vi "ExampleVI.vi"() -> ()   [LabVIEW 2024]
uses:
  DeconEngineClass/LaguerreDeconEngineClass.lvclass
  DeconEngineClass/LaguerreDeconEngineClass.lvclass/LaguerreDeconEngineClass.ctl
  <vilib>/Analysis/baseanly.llb/Mean (DBL).vi
  <vilib>/Utility/file.llb/Read Delimited Spreadsheet (DBL).vi
  <vilib>/Analysis/NI_AALBase.lvlib
panel:
  out "Histogram Graph":T1(graph)
  out "Lifetime Graph":dbl[](graph)
  out "iRF shift":dbl
  out "RMSE":dbl[](array[numeric])
  out "R square":dbl[](array[numeric])
  out "SSE":dbl[](array[numeric])
  in  "dataLength":i32=680
  out "iRF size(s)":i32
  out "data Matrix Szie":T2
  in  "plot index (row)":i32=45
  out "Decay Graph":dbl[][](graph)
  out "Computer time Graph":dbl[](graph)
  out "data Length":i32
  out "Waveform Graph":dbl[][](graph)
  out "alpha value":dbl
  in  "LaguerreDeconLib.lvlib:LaguerreDeconClass.lvclass":refnum<class "LaguerreDeconEngineClass.lvclass">
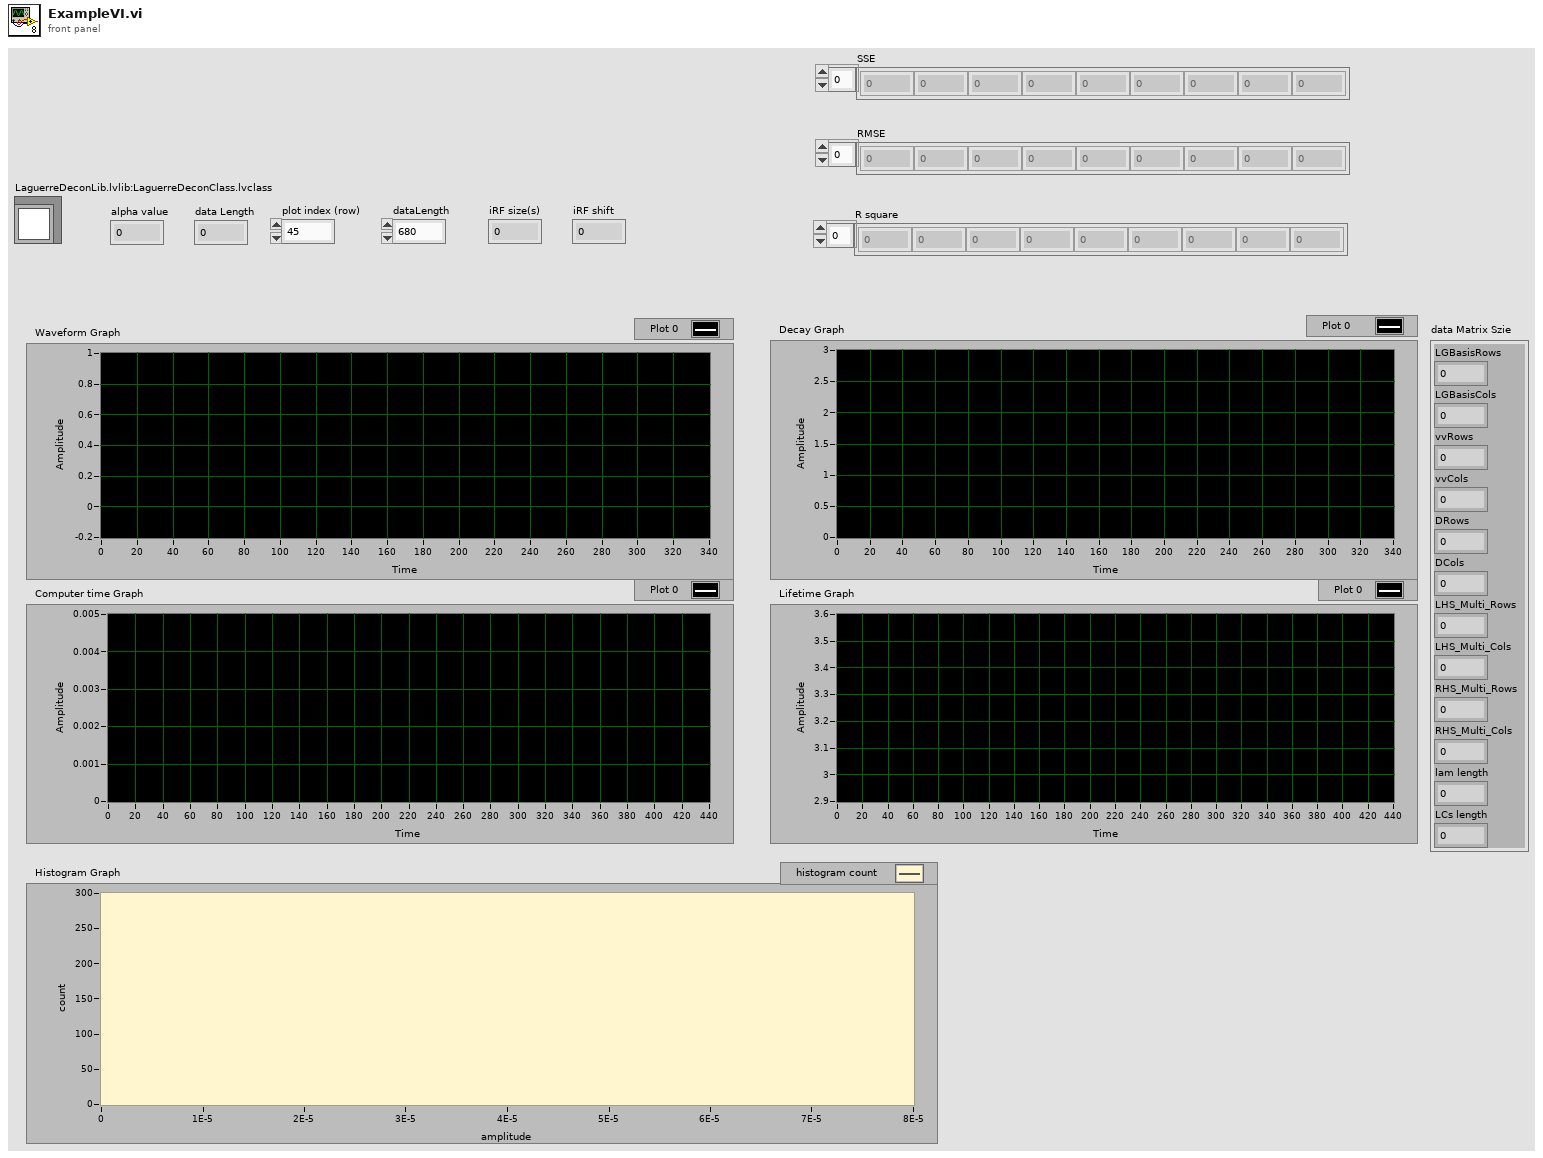
[diagram p1: front panel]
types:
  T1 = cluster{"X Values":dbl[], "Histogram: h(x)":i32[]}
  T2 = cluster{"LGBasisRows":u32, "LGBasisCols":u32, "vvRows":u32, "vvCols":u32, "DRows":u32, "DCols":u32, "LHS_Multi_Rows":u32, "LHS_Multi_Cols":u32, "RHS_Multi_Rows":u32, "RHS_Multi_Cols":u32, "lam length":u32, "LCs length":u32}
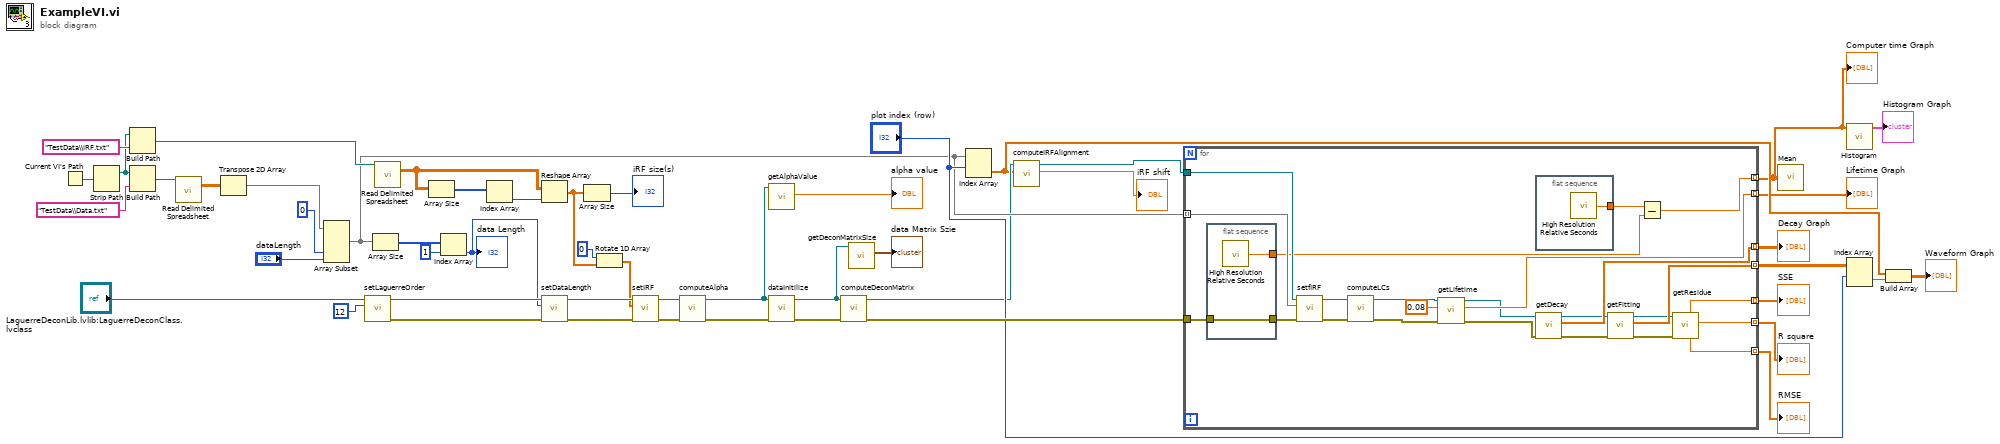
[diagram p0: block diagram]
diagram:
  n1 = Current VI's Path() -> (path=w22:path)
  n2 = Strip Path(path=w22) -> (stripped path=w18:path)  [unwired: 1 out]
  n3 = Build Path(base path=w18, name or relative path="TestData\\iRF.txt") -> (appended path=w17:path)
  n4 = Build Path(base path=w18, name or relative path="TestData\\Data.txt") -> (appended path=w20:path)
  n5 = call-poly <vilib>:"Read Delimited Spreadsheet.vi"("file path (dialog if empty)"=w20) -> ("all rows"=w35:dbl[][])  [unwired: 9 in, 5 out]
  n6 = Transpose 2D Array(2D array=w35) -> (transposed array=w33:dbl[][])
  n7 = Array Subset(array=w33, index (col)=0 ("index"), length (col)="dataLength") -> (w11:dbl[][])  [unwired: 2 in]
  n8 = call "setLaguerreOrder.vi"("LaguerreOrder"=u64 12, "LaguerreDeconClass in"="LaguerreDeconLib.lvlib:LaguerreDeconClass.lvclass") -> ("error out"=w46:errorcluster, "LaguerreDeconClass out"=w47:refnum<class "LaguerreDeconEngineClass.lvclass">)  [unwired: 8 in]
  n9 = Array Size(array=w11) -> (size(s)=w37:i32[])
  n10 = call-poly <vilib>:"Read Delimited Spreadsheet.vi"("file path (dialog if empty)"=w17) -> ("all rows"=w50:dbl[][])  [unwired: 9 in, 5 out]
  n11 = Array Size(array=w50) -> (size(s)=w51:i32[])
  n12 = Index Array(array=w37, index=1) -> (element=w36:i32)
  "data Length" <- w36
  n13 = Index Array(array=w51) -> (element=w40:i32)  [unwired: 1 in]
  n14 = Reshape Array(w50, w40) -> (w9:dbl[])
  n15 = call "setDataLength.vi"("error in (no error)"=w46, "dataLength"=w36, "LaguerreDeconClass in"=w47) -> ("error out"=w44:errorcluster, "LaguerreDeconClass out"=w45:refnum<class "LaguerreDeconEngineClass.lvclass">)  [unwired: 7 in]
  n16 = Array Size(array=w9) -> (size(s)=→"iRF size(s)":i32)
  n17 = Rotate 1D Array(1:w9, 2:0 ("n")) -> (0:w8:dbl[])
  n18 = call "setIRF.vi"("error in (no error)"=w44, "iRF"=w8, "LaguerreDeconClass in"=w45) -> ("error out"=w42:errorcluster, "LaguerreDeconClass out"=w43:refnum<class "LaguerreDeconEngineClass.lvclass">)  [unwired: 7 in]
  n19 = call "computeAlpha.vi"("error in (no error)"=w42, "LaguerreDeconClass in"=w43) -> ("error out"=w41:errorcluster, "LaguerreDeconClass out"=w30:refnum<class "LaguerreDeconEngineClass.lvclass">)  [unwired: 8 in]
  n20 = call "getAlphaValue.vi"("LaguerreDeconClass in"=w30) -> ("alpha value"=→"alpha value":dbl)  [unwired: 8 in, 2 out]
  n21 = call "dataInitilize.vi"("error in (no error)"=w41, "LaguerreDeconClass in"=w30) -> ("error out"=w39:errorcluster, "LaguerreDeconClass out"=w25:refnum<class "LaguerreDeconEngineClass.lvclass">)  [unwired: 8 in]
  n22 = call "computeDeconMatrix.vi"("error in (no error)"=w39, "LaguerreDeconClass in"=w25) -> ("error out"=w38:errorcluster, "LaguerreDeconClass out"=w10:refnum<class "LaguerreDeconEngineClass.lvclass">)  [unwired: 8 in]
  n23 = call "getDeconMatrixSize.vi"("LaguerreDeconClass in"=w25) -> ("data Matrix Szie"=→"data Matrix Szie":T2)  [unwired: 8 in, 2 out]
  n24 = Index Array(array=w11, index (row)="plot index (row)") -> (element=w5:dbl[])  [unwired: 1 in]
  n25 = call "computeIRFAlignment.vi"("fIRF temp"=w5, "LaguerreDeconEngineClass in"=w10) -> ("iRF shift"=→"iRF shift":dbl, "LaguerreDeconEngineClass out"=w4:refnum<class "LaguerreDeconEngineClass.lvclass">)  [unwired: 7 in, 1 out]
  n26 = for {
    tunnel: w4 -> [w70]
    tunnel: w38 -> [w58]
    tunnel: w11 -> [w68] mode=indexing
    tunnel: [w74] -> w2 mode=indexing
    tunnel: [w73] -> w31 mode=indexing
    tunnel: [w71] -> w28 mode=indexing
    tunnel: [w65] -> w14 mode=indexing
    tunnel: [w64] -> w13 mode=indexing
    tunnel: [w63] -> w12 mode=indexing
    tunnel: [w62] -> w3 mode=indexing
    n27 = flat-sequence {
      tunnel: [w77] -> w60
      tunnel: w58 -> [w76]
      tunnel: [w76] -> w57
      frame #0 {
        n28 = call <vilib>:"High Resolution Relative Seconds.vi"() -> ("relative seconds"=w77:dbl)
      }
    }
    n29 = call "setfIRF.vi"("error in (no error)"=w57, "fIRF"=w68, "LaguerreDeconEngineClass in"=w70) -> ("error out"=w59:errorcluster, "LaguerreDeconEngineClass out"=w69:refnum<class "LaguerreDeconEngineClass.lvclass">)  [unwired: 7 in]
    n30 = call "computeLCs.vi"("error in (no error)"=w59, "LaguerreDeconClass in"=w69) -> ("error out"=w55:errorcluster, "LaguerreDeconClass out"=w54:refnum<class "LaguerreDeconEngineClass.lvclass">)  [unwired: 8 in]
    n31 = call "getLifetime.vi"("error in (no error)"=w55, "dt (ns)"=0.08, "LaguerreDeconEngineClass in"=w54) -> ("error out"=w52:errorcluster, "lifetime (ns)"=w62:dbl, "LaguerreDeconEngineClass out"=w53:refnum<class "LaguerreDeconEngineClass.lvclass">)  [unwired: 6 in]
    n32 = flat-sequence {
      tunnel: [w78] -> w75
      frame #0 {
        n33 = call <vilib>:"High Resolution Relative Seconds.vi"() -> ("relative seconds"=w78:dbl)
      }
    }
    n34 = call "getDecay.vi"("error in (no error)"=w52, "LaguerreDeconClass in"=w53) -> ("error out"=w56:errorcluster, "Decay"=w73:dbl[], "LaguerreDeconClass out"=w72:refnum<class "LaguerreDeconEngineClass.lvclass">)  [unwired: 7 in]
    n35 = call "getFitting.vi"("error in (no error)"=w56, "LaguerreDeconEngineClass in"=w72) -> ("error out"=w66:errorcluster, "Fitting"=w71:dbl[], "LaguerreDeconEngineClass out"=w67:refnum<class "LaguerreDeconEngineClass.lvclass">)  [unwired: 7 in]
    n36 = Subtract(x=w75, y=w60) -> (x-y=w74:dbl)
    n37 = call "getResidue.vi"("error in (no error)"=w66, "LaguerreDeconEngineClass in"=w67) -> ("R-square"=w64:dbl, "RMSE"=w63:dbl, "SSE"=w65:dbl)  [unwired: 5 in, 2 out]
  }
  "Computer time Graph" <- w2
  "Decay Graph" <- w31
  "SSE" <- w14
  "R square" <- w13
  "RMSE" <- w12
  "Lifetime Graph" <- w3
  n38 = call-poly <vilib>:"Mean.vi"("X"=w2) -> ()  [unwired: 2 out]
  n39 = call <vilib>:"Histogram.vi"("X"=w2) -> ("Histogram Graph"=→"Histogram Graph":T1)  [unwired: 7 in, 3 out]
  n40 = Index Array(array=w28, index (row)="plot index (row)") -> (element=w27:dbl[])  [unwired: 1 in]
  n41 = Build Array(w5, w27) -> (→"Waveform Graph":dbl[][])
